vi "Write Index.vi"(8 "error in (no error)":errorcluster, 10 "Index":i32, 11 "GenericDevice in":refnum<class "GenericDevice.lvclass">) -> (0 "error out":errorcluster, 3 "GenericDevice out":refnum<class "GenericDevice.lvclass">)   [LabVIEW 2020, in "horiba.lvlib" / "GenericDevice.lvclass"]
doc: "Accessor VI for this class property."
uses:
  GenericDevice.lvclass
  GenericDevice.lvclass/GenericDevice.ctl
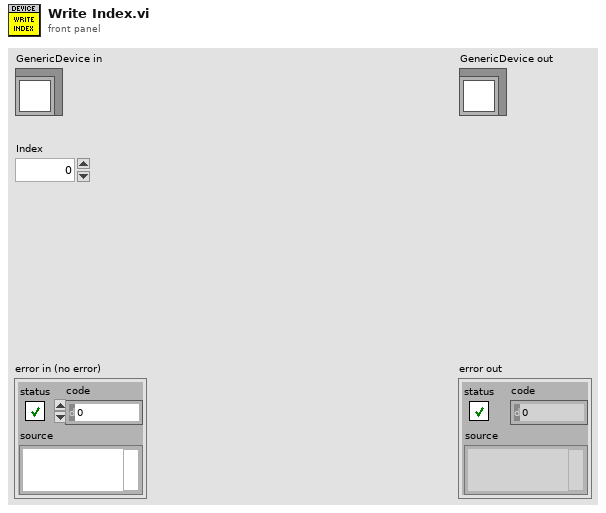
[diagram p1: front panel]
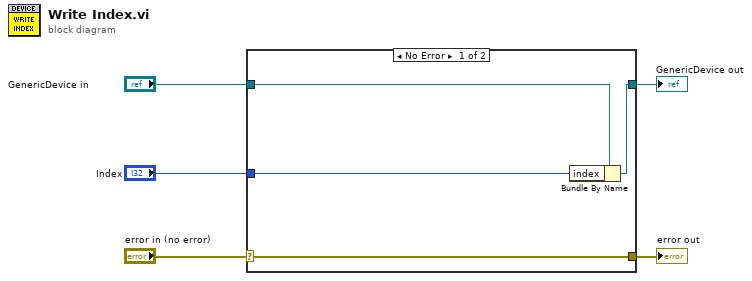
[diagram p0: block diagram]
diagram:
  n1 = case shown="No Error" "error in (no error)" {
    selector: "error in (no error)" -> [w9 w10]
    tunnel: [w9 w10] -> w4
    tunnel: [w7 w11] -> w2
    tunnel: "GenericDevice in" -> [w8 w11]
    tunnel: "Index" -> [w6 _]
    frame No Error {
      n2 = Bundle By Name(cluster=w8, "index"=w6) -> (w7:refnum<class "GenericDevice.lvclass">)
    }
    frame Error {
    }
  }
  "error out" <- w4
  "GenericDevice out" <- w2
